vi "RtdeGetLatestOutputValues.vi"(8 "Rtde":refnum<k24>, 11 "error in":errorcluster) -> (0 "Data":T1, 3 "error out":errorcluster)   [LabVIEW 2015, in "UnderAutomation.UniversalRobots.lvlib"]
uses:
  UnderAutomation.UniversalRobots.lvlib
  C:/Users/fg/Documents/UniversalRobots.vi/LabVIEW_2024/UnderAutomation.UniversalRobots/lib/UnderAutomation.UniversalRobots.dll
  LabVIEW_2024/UnderAutomation.UniversalRobots/lib/UnderAutomation.UniversalRobots.dll
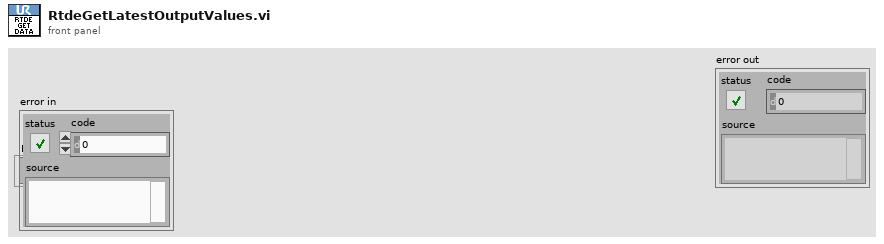
[diagram p1: front panel]
types:
  T1 = cluster{"ActualCurrent":cluster{"Base":dbl, "Elbow":dbl, "Shoulder":dbl, "Wrist1":dbl, "Wrist2":dbl, "Wrist3":dbl}, "ActualDigitalInputBits":u64, "ActualDigitalOutputBits":u64, "ActualExecutionTime":dbl, "ActualJointVoltage":cluster{"Base":dbl, "Elbow":dbl, "Shoulder":dbl, "Wrist1":dbl, "Wrist2":dbl, "Wrist3":dbl}, "ActualMainVoltage":dbl, "ActualMomentum":dbl, "ActualQ":cluster{"Base":dbl, "Elbow":dbl, "Shoulder":dbl, "Wrist1":dbl, "Wrist2":dbl, "Wrist3":dbl}, "ActualQd":cluster{"Base":dbl, "Elbow":dbl, "Shoulder":dbl, "Wrist1":dbl, "Wrist2":dbl, "Wrist3":dbl}, "ActualRobotCurrent":dbl, "ActualRobotVoltage":dbl, "ActualTcpForce":cluster{"X":dbl, "Y":dbl, "Z":dbl, "Rx":dbl, "Ry":dbl, "Rz":dbl}, "ActualTcpPose":cluster{"X":dbl, "Y":dbl, "Z":dbl, "Rx":dbl, "Ry":dbl, "Rz":dbl}, "ActualTcpSpeed":cluster{"X":dbl, "Y":dbl, "Z":dbl, "Rx":dbl, "Ry":dbl, "Rz":dbl}, "ActualToolAccelerometer":cluster{"X":dbl, "Y":dbl, "Z":dbl}, "AnalogIOTypes":u32, "ElbowPosition":cluster{"X":dbl, "Y":dbl, "Z":dbl}, "ElbowVelocity":cluster{"X":dbl, "Y":dbl, "Z":dbl}, "Euromap67_24VCurrent":dbl, "Euromap67_24VVoltage":dbl, "Euromap67InputBits":u32, "Euromap67OutputBits":u32, "FTRawWrench":cluster{"X":dbl, "Y":dbl, "Z":dbl, "Rx":dbl, "Ry":dbl, "Rz":dbl}, "InputBitRegisters":cluster{"X64":bool, "X65":bool, "X66":bool, "X67":bool, "X68":bool, "X69":bool, "X70":bool, "X71":bool, "X72":bool, "X73":bool, "X74":bool, "X75":bool, "X76":bool, "X77":bool, "X78":bool, "X79":bool, "X80":bool, "X81":bool, "X82":bool, "X83":bool, "X84":bool, "X85":bool, "X86":bool, "X87":bool, "X88":bool, "X89":bool, "X90":bool, "X91":bool, "X92":bool, "X93":bool, "X94":bool, "X95":bool, "X96":bool, "X97":bool, "X98":bool, "X99":bool, "X100":bool, "X101":bool, "X102":bool, "X103":bool, "X104":bool, "X105":bool, "X106":bool, "X107":bool, "X108":bool, "X109":bool, "X110":bool, "X111":bool, "X112":bool, "X113":bool, "X114":bool, "X115":bool, "X116":bool, "X117":bool, "X118":bool, "X119":bool, "X120":bool, "X121":bool, "X122":bool, "X123":bool, "X124":bool, "X125":bool, "X126":bool, "X127":bool}, "InputBitRegisters0To31":u32, "InputBitRegisters32To63":u32, "InputDoubleRegisters":cluster{"X0":dbl, "X1":dbl, "X2":dbl, "X3":dbl, "X4":dbl, "X5":dbl, "X6":dbl, "X7":dbl, "X8":dbl, "X9":dbl, "X10":dbl, "X11":dbl, "X12":dbl, "X13":dbl, "X14":dbl, "X15":dbl, "X16":dbl, "X17":dbl, "X18":dbl, "X19":dbl, "X20":dbl, "X21":dbl, "X22":dbl, "X23":dbl, "X24":dbl, "X25":dbl, "X26":dbl, "X27":dbl, "X28":dbl, "X29":dbl, "X30":dbl, "X31":dbl, "X32":dbl, "X33":dbl, "X34":dbl, "X35":dbl, "X36":dbl, "X37":dbl, "X38":dbl, "X39":dbl, "X40":dbl, "X41":dbl, "X42":dbl, "X43":dbl, "X44":dbl, "X45":dbl, "X46":dbl, "X47":dbl}, "InputIntRegisters":cluster{"X0":i32, "X1":i32, "X2":i32, "X3":i32, "X4":i32, "X5":i32, "X6":i32, "X7":i32, "X8":i32, "X9":i32, "X10":i32, "X11":i32, "X12":i32, "X13":i32, "X14":i32, "X15":i32, "X16":i32, "X17":i32, "X18":i32, "X19":i32, "X20":i32, "X21":i32, "X22":i32, "X23":i32, "X24":i32, "X25":i32, "X26":i32, "X27":i32, "X28":i32, "X29":i32, "X30":i32, "X31":i32, "X32":i32, "X33":i32, "X34":i32, "X35":i32, "X36":i32, "X37":i32, "X38":i32, "X39":i32, "X40":i32, "X41":i32, "X42":i32, "X43":i32, "X44":i32, "X45":i32, "X46":i32, "X47":i32}, "IOCurrent":dbl, "JointControlOutput":cluster{"Base":dbl, "Elbow":dbl, "Shoulder":dbl, "Wrist1":dbl, "Wrist2":dbl, "Wrist3":dbl}, "JointMode":cluster{"Base":i32, "Elbow":i32, "Shoulder":i32, "Wrist1":i32, "Wrist2":i32, "Wrist3":i32}, "JointTemperatures":cluster{"Base":dbl, "Elbow":dbl, "Shoulder":dbl, "Wrist1":dbl, "Wrist2":dbl, "Wrist3":dbl}, "OutputBitRegisters":cluster{"X64":bool, "X65":bool, "X66":bool, "X67":bool, "X68":bool, "X69":bool, "X70":bool, "X71":bool, "X72":bool, "X73":bool, "X74":bool, "X75":bool, "X76":bool, "X77":bool, "X78":bool, "X79":bool, "X80":bool, "X81":bool, "X82":bool, "X83":bool, "X84":bool, "X85":bool, "X86":bool, "X87":bool, "X88":bool, "X89":bool, "X90":bool, "X91":bool, "X92":bool, "X93":bool, "X94":bool, "X95":bool, "X96":bool, "X97":bool, "X98":bool, "X99":bool, "X100":bool, "X101":bool, "X102":bool, "X103":bool, "X104":bool, "X105":bool, "X106":bool, "X107":bool, "X108":bool, "X109":bool, "X110":bool, "X111":bool, "X112":bool, "X113":bool, "X114":bool, "X115":bool, "X116":bool, "X117":bool, "X118":bool, "X119":bool, "X120":bool, "X121":bool, "X122":bool, "X123":bool, "X124":bool, "X125":bool, "X126":bool, "X127":bool}, "OutputBitRegisters0To31":u32, "OutputBitRegisters32To63":u32, "OutputDoubleRegisters":cluster{"X0":dbl, "X1":dbl, "X2":dbl, "X3":dbl, "X4":dbl, "X5":dbl, "X6":dbl, "X7":dbl, "X8":dbl, "X9":dbl, "X10":dbl, "X11":dbl, "X12":dbl, "X13":dbl, "X14":dbl, "X15":dbl, "X16":dbl, "X17":dbl, "X18":dbl, "X19":dbl, "X20":dbl, "X21":dbl, "X22":dbl, "X23":dbl, "X24":dbl, "X25":dbl, "X26":dbl, "X27":dbl, "X28":dbl, "X29":dbl, "X30":dbl, "X31":dbl, "X32":dbl, "X33":dbl, "X34":dbl, "X35":dbl, "X36":dbl, "X37":dbl, "X38":dbl, "X39":dbl, "X40":dbl, "X41":dbl, "X42":dbl, "X43":dbl, "X44":dbl, "X45":dbl, "X46":dbl, "X47":dbl}, "OutputIntRegisters":cluster{"X0":i32, "X1":i32, "X2":i32, "X3":i32, "X4":i32, "X5":i32, "X6":i32, "X7":i32, "X8":i32, "X9":i32, "X10":i32, "X11":i32, "X12":i32, "X13":i32, "X14":i32, "X15":i32, "X16":i32, "X17":i32, "X18":i32, "X19":i32, "X20":i32, "X21":i32, "X22":i32, "X23":i32, "X24":i32, "X25":i32, "X26":i32, "X27":i32, "X28":i32, "X29":i32, "X30":i32, "X31":i32, "X32":i32, "X33":i32, "X34":i32, "X35":i32, "X36":i32, "X37":i32, "X38":i32, "X39":i32, "X40":i32, "X41":i32, "X42":i32, "X43":i32, "X44":i32, "X45":i32, "X46":i32, "X47":i32}, "Payload":dbl, "PayloadCOG":cluster{"X":dbl, "Y":dbl, "Z":dbl}, "PayloadInertia":cluster{"X":dbl, "Y":dbl, "Z":dbl, "Rx":dbl, "Ry":dbl, "Rz":dbl}, "RobotMode":i32, "RobotStatusBits":u32, "RuntimeState":u32, "SafetyMode":i32, "SafetyStatus":i32, "SafetyStatusBits":u32, "ScriptControlLine":u32, "SpeedScaling":dbl, "StandardAnalogInput0":dbl, "StandardAnalogInput1":dbl, "StandardAnalogOutput0":dbl, "StandardAnalogOutput1":dbl, "TargetCurrent":cluster{"Base":dbl, "Elbow":dbl, "Shoulder":dbl, "Wrist1":dbl, "Wrist2":dbl, "Wrist3":dbl}, "TargetMoment":cluster{"Base":dbl, "Elbow":dbl, "Shoulder":dbl, "Wrist1":dbl, "Wrist2":dbl, "Wrist3":dbl}, "TargetQ":cluster{"Base":dbl, "Elbow":dbl, "Shoulder":dbl, "Wrist1":dbl, "Wrist2":dbl, "Wrist3":dbl}, "TargetQd":cluster{"Base":dbl, "Elbow":dbl, "Shoulder":dbl, "Wrist1":dbl, "Wrist2":dbl, "Wrist3":dbl}, "TargetQdd":cluster{"Base":dbl, "Elbow":dbl, "Shoulder":dbl, "Wrist1":dbl, "Wrist2":dbl, "Wrist3":dbl}, "TargetSpeedFraction":dbl, "TargetTcpPose":cluster{"X":dbl, "Y":dbl, "Z":dbl, "Rx":dbl, "Ry":dbl, "Rz":dbl}, "TargetTcpSpeed":cluster{"X":dbl, "Y":dbl, "Z":dbl, "Rx":dbl, "Ry":dbl, "Rz":dbl}, "TcpForceScalar":dbl, "Timestamp":dbl, "ToolAnalogInput0":dbl, "ToolAnalogInput1":dbl, "ToolAnalogInputTypes":u32, "ToolDigitalOutput0mode":u8, "ToolDigitalOutput1Mode":u8, "ToolMode":u32, "ToolOutputCurrent":dbl, "ToolOutputMode":u8, "ToolOutputVoltage":i32, "ToolTemperature":dbl}
  T2 = cluster{"Base":dbl, "Elbow":dbl, "Shoulder":dbl, "Wrist1":dbl, "Wrist2":dbl, "Wrist3":dbl}
  T3 = cluster{"X":dbl, "Y":dbl, "Z":dbl, "Rx":dbl, "Ry":dbl, "Rz":dbl}
  T4 = cluster{"X64":bool, "X65":bool, "X66":bool, "X67":bool, "X68":bool, "X69":bool, "X70":bool, "X71":bool, "X72":bool, "X73":bool, "X74":bool, "X75":bool, "X76":bool, "X77":bool, "X78":bool, "X79":bool, "X80":bool, "X81":bool, "X82":bool, "X83":bool, "X84":bool, "X85":bool, "X86":bool, "X87":bool, "X88":bool, "X89":bool, "X90":bool, "X91":bool, "X92":bool, "X93":bool, "X94":bool, "X95":bool, "X96":bool, "X97":bool, "X98":bool, "X99":bool, "X100":bool, "X101":bool, "X102":bool, "X103":bool, "X104":bool, "X105":bool, "X106":bool, "X107":bool, "X108":bool, "X109":bool, "X110":bool, "X111":bool, "X112":bool, "X113":bool, "X114":bool, "X115":bool, "X116":bool, "X117":bool, "X118":bool, "X119":bool, "X120":bool, "X121":bool, "X122":bool, "X123":bool, "X124":bool, "X125":bool, "X126":bool, "X127":bool}
  T5 = cluster{"X0":dbl, "X1":dbl, "X2":dbl, "X3":dbl, "X4":dbl, "X5":dbl, "X6":dbl, "X7":dbl, "X8":dbl, "X9":dbl, "X10":dbl, "X11":dbl, "X12":dbl, "X13":dbl, "X14":dbl, "X15":dbl, "X16":dbl, "X17":dbl, "X18":dbl, "X19":dbl, "X20":dbl, "X21":dbl, "X22":dbl, "X23":dbl, "X24":dbl, "X25":dbl, "X26":dbl, "X27":dbl, "X28":dbl, "X29":dbl, "X30":dbl, "X31":dbl, "X32":dbl, "X33":dbl, "X34":dbl, "X35":dbl, "X36":dbl, "X37":dbl, "X38":dbl, "X39":dbl, "X40":dbl, "X41":dbl, "X42":dbl, "X43":dbl, "X44":dbl, "X45":dbl, "X46":dbl, "X47":dbl}
  T6 = cluster{"Base":i32, "Elbow":i32, "Shoulder":i32, "Wrist1":i32, "Wrist2":i32, "Wrist3":i32}
  T7 = cluster{"X0":i32, "X1":i32, "X2":i32, "X3":i32, "X4":i32, "X5":i32, "X6":i32, "X7":i32, "X8":i32, "X9":i32, "X10":i32, "X11":i32, "X12":i32, "X13":i32, "X14":i32, "X15":i32, "X16":i32, "X17":i32, "X18":i32, "X19":i32, "X20":i32, "X21":i32, "X22":i32, "X23":i32, "X24":i32, "X25":i32, "X26":i32, "X27":i32, "X28":i32, "X29":i32, "X30":i32, "X31":i32, "X32":i32, "X33":i32, "X34":i32, "X35":i32, "X36":i32, "X37":i32, "X38":i32, "X39":i32, "X40":i32, "X41":i32, "X42":i32, "X43":i32, "X44":i32, "X45":i32, "X46":i32, "X47":i32}
  T8 = cluster{cluster{"Base":dbl, "Elbow":dbl, "Shoulder":dbl, "Wrist1":dbl, "Wrist2":dbl, "Wrist3":dbl}, "ActualDigitalInputBits":u64, "ActualDigitalOutputBits":u64, "ActualExecutionTime":dbl, cluster{"Base":dbl, "Elbow":dbl, "Shoulder":dbl, "Wrist1":dbl, "Wrist2":dbl, "Wrist3":dbl}, "ActualMainVoltage":dbl, "ActualMomentum":dbl, cluster{"Base":dbl, "Elbow":dbl, "Shoulder":dbl, "Wrist1":dbl, "Wrist2":dbl, "Wrist3":dbl}, cluster{"Base":dbl, "Elbow":dbl, "Shoulder":dbl, "Wrist1":dbl, "Wrist2":dbl, "Wrist3":dbl}, "ActualRobotCurrent":dbl, "ActualRobotVoltage":dbl, cluster{"X":dbl, "Y":dbl, "Z":dbl, "Rx":dbl, "Ry":dbl, "Rz":dbl}, cluster{"X":dbl, "Y":dbl, "Z":dbl, "Rx":dbl, "Ry":dbl, "Rz":dbl}, cluster{"X":dbl, "Y":dbl, "Z":dbl, "Rx":dbl, "Ry":dbl, "Rz":dbl}, cluster{"X":dbl, "Y":dbl, "Z":dbl}, "AnalogIOTypes":u32, cluster{"X":dbl, "Y":dbl, "Z":dbl}, cluster{"X":dbl, "Y":dbl, "Z":dbl}, "Euromap67_24VCurrent":dbl, "Euromap67_24VVoltage":dbl, "Euromap67InputBits":u32, "Euromap67OutputBits":u32, cluster{"X":dbl, "Y":dbl, "Z":dbl, "Rx":dbl, "Ry":dbl, "Rz":dbl}, cluster{"X64":bool, "X65":bool, "X66":bool, "X67":bool, "X68":bool, "X69":bool, "X70":bool, "X71":bool, "X72":bool, "X73":bool, "X74":bool, "X75":bool, "X76":bool, "X77":bool, "X78":bool, "X79":bool, "X80":bool, "X81":bool, "X82":bool, "X83":bool, "X84":bool, "X85":bool, "X86":bool, "X87":bool, "X88":bool, "X89":bool, "X90":bool, "X91":bool, "X92":bool, "X93":bool, "X94":bool, "X95":bool, "X96":bool, "X97":bool, "X98":bool, "X99":bool, "X100":bool, "X101":bool, "X102":bool, "X103":bool, "X104":bool, "X105":bool, "X106":bool, "X107":bool, "X108":bool, "X109":bool, "X110":bool, "X111":bool, "X112":bool, "X113":bool, "X114":bool, "X115":bool, "X116":bool, "X117":bool, "X118":bool, "X119":bool, "X120":bool, "X121":bool, "X122":bool, "X123":bool, "X124":bool, "X125":bool, "X126":bool, "X127":bool}, "InputBitRegisters0To31":u32, "InputBitRegisters32To63":u32, cluster{"X0":dbl, "X1":dbl, "X2":dbl, "X3":dbl, "X4":dbl, "X5":dbl, "X6":dbl, "X7":dbl, "X8":dbl, "X9":dbl, "X10":dbl, "X11":dbl, "X12":dbl, "X13":dbl, "X14":dbl, "X15":dbl, "X16":dbl, "X17":dbl, "X18":dbl, "X19":dbl, "X20":dbl, "X21":dbl, "X22":dbl, "X23":dbl, "X24":dbl, "X25":dbl, "X26":dbl, "X27":dbl, "X28":dbl, "X29":dbl, "X30":dbl, "X31":dbl, "X32":dbl, "X33":dbl, "X34":dbl, "X35":dbl, "X36":dbl, "X37":dbl, "X38":dbl, "X39":dbl, "X40":dbl, "X41":dbl, "X42":dbl, "X43":dbl, "X44":dbl, "X45":dbl, "X46":dbl, "X47":dbl}, cluster{"X0":i32, "X1":i32, "X2":i32, "X3":i32, "X4":i32, "X5":i32, "X6":i32, "X7":i32, "X8":i32, "X9":i32, "X10":i32, "X11":i32, "X12":i32, "X13":i32, "X14":i32, "X15":i32, "X16":i32, "X17":i32, "X18":i32, "X19":i32, "X20":i32, "X21":i32, "X22":i32, "X23":i32, "X24":i32, "X25":i32, "X26":i32, "X27":i32, "X28":i32, "X29":i32, "X30":i32, "X31":i32, "X32":i32, "X33":i32, "X34":i32, "X35":i32, "X36":i32, "X37":i32, "X38":i32, "X39":i32, "X40":i32, "X41":i32, "X42":i32, "X43":i32, "X44":i32, "X45":i32, "X46":i32, "X47":i32}, "IOCurrent":dbl, cluster{"Base":dbl, "Elbow":dbl, "Shoulder":dbl, "Wrist1":dbl, "Wrist2":dbl, "Wrist3":dbl}, cluster{"Base":i32, "Elbow":i32, "Shoulder":i32, "Wrist1":i32, "Wrist2":i32, "Wrist3":i32}, cluster{"Base":dbl, "Elbow":dbl, "Shoulder":dbl, "Wrist1":dbl, "Wrist2":dbl, "Wrist3":dbl}, cluster{"X64":bool, "X65":bool, "X66":bool, "X67":bool, "X68":bool, "X69":bool, "X70":bool, "X71":bool, "X72":bool, "X73":bool, "X74":bool, "X75":bool, "X76":bool, "X77":bool, "X78":bool, "X79":bool, "X80":bool, "X81":bool, "X82":bool, "X83":bool, "X84":bool, "X85":bool, "X86":bool, "X87":bool, "X88":bool, "X89":bool, "X90":bool, "X91":bool, "X92":bool, "X93":bool, "X94":bool, "X95":bool, "X96":bool, "X97":bool, "X98":bool, "X99":bool, "X100":bool, "X101":bool, "X102":bool, "X103":bool, "X104":bool, "X105":bool, "X106":bool, "X107":bool, "X108":bool, "X109":bool, "X110":bool, "X111":bool, "X112":bool, "X113":bool, "X114":bool, "X115":bool, "X116":bool, "X117":bool, "X118":bool, "X119":bool, "X120":bool, "X121":bool, "X122":bool, "X123":bool, "X124":bool, "X125":bool, "X126":bool, "X127":bool}, "OutputBitRegisters0To31":u32, "OutputBitRegisters32To63":u32, cluster{"X0":dbl, "X1":dbl, "X2":dbl, "X3":dbl, "X4":dbl, "X5":dbl, "X6":dbl, "X7":dbl, "X8":dbl, "X9":dbl, "X10":dbl, "X11":dbl, "X12":dbl, "X13":dbl, "X14":dbl, "X15":dbl, "X16":dbl, "X17":dbl, "X18":dbl, "X19":dbl, "X20":dbl, "X21":dbl, "X22":dbl, "X23":dbl, "X24":dbl, "X25":dbl, "X26":dbl, "X27":dbl, "X28":dbl, "X29":dbl, "X30":dbl, "X31":dbl, "X32":dbl, "X33":dbl, "X34":dbl, "X35":dbl, "X36":dbl, "X37":dbl, "X38":dbl, "X39":dbl, "X40":dbl, "X41":dbl, "X42":dbl, "X43":dbl, "X44":dbl, "X45":dbl, "X46":dbl, "X47":dbl}, cluster{"X0":i32, "X1":i32, "X2":i32, "X3":i32, "X4":i32, "X5":i32, "X6":i32, "X7":i32, "X8":i32, "X9":i32, "X10":i32, "X11":i32, "X12":i32, "X13":i32, "X14":i32, "X15":i32, "X16":i32, "X17":i32, "X18":i32, "X19":i32, "X20":i32, "X21":i32, "X22":i32, "X23":i32, "X24":i32, "X25":i32, "X26":i32, "X27":i32, "X28":i32, "X29":i32, "X30":i32, "X31":i32, "X32":i32, "X33":i32, "X34":i32, "X35":i32, "X36":i32, "X37":i32, "X38":i32, "X39":i32, "X40":i32, "X41":i32, "X42":i32, "X43":i32, "X44":i32, "X45":i32, "X46":i32, "X47":i32}, "Payload":dbl, cluster{"X":dbl, "Y":dbl, "Z":dbl}, cluster{"X":dbl, "Y":dbl, "Z":dbl, "Rx":dbl, "Ry":dbl, "Rz":dbl}, "RobotMode":i32, "RobotStatusBits":u32, "RuntimeState":u32, "SafetyMode":i32, "SafetyStatus":i32, "SafetyStatusBits":u32, "ScriptControlLine":u32, "SpeedScaling":dbl, "StandardAnalogInput0":dbl, "StandardAnalogInput1":dbl, "StandardAnalogOutput0":dbl, "StandardAnalogOutput1":dbl, cluster{"Base":dbl, "Elbow":dbl, "Shoulder":dbl, "Wrist1":dbl, "Wrist2":dbl, "Wrist3":dbl}, cluster{"Base":dbl, "Elbow":dbl, "Shoulder":dbl, "Wrist1":dbl, "Wrist2":dbl, "Wrist3":dbl}, cluster{"Base":dbl, "Elbow":dbl, "Shoulder":dbl, "Wrist1":dbl, "Wrist2":dbl, "Wrist3":dbl}, cluster{"Base":dbl, "Elbow":dbl, "Shoulder":dbl, "Wrist1":dbl, "Wrist2":dbl, "Wrist3":dbl}, cluster{"Base":dbl, "Elbow":dbl, "Shoulder":dbl, "Wrist1":dbl, "Wrist2":dbl, "Wrist3":dbl}, "TargetSpeedFraction":dbl, cluster{"X":dbl, "Y":dbl, "Z":dbl, "Rx":dbl, "Ry":dbl, "Rz":dbl}, cluster{"X":dbl, "Y":dbl, "Z":dbl, "Rx":dbl, "Ry":dbl, "Rz":dbl}, "TcpForceScalar":dbl, "Timestamp":dbl, "ToolAnalogInput0":dbl, "ToolAnalogInput1":dbl, "ToolAnalogInputTypes":u32, "ToolDigitalOutput0mode":u8, "ToolDigitalOutput1Mode":u8, "ToolMode":u32, "ToolOutputCurrent":dbl, "ToolOutputMode":u8, "ToolOutputVoltage":i32, "ToolTemperature":dbl}
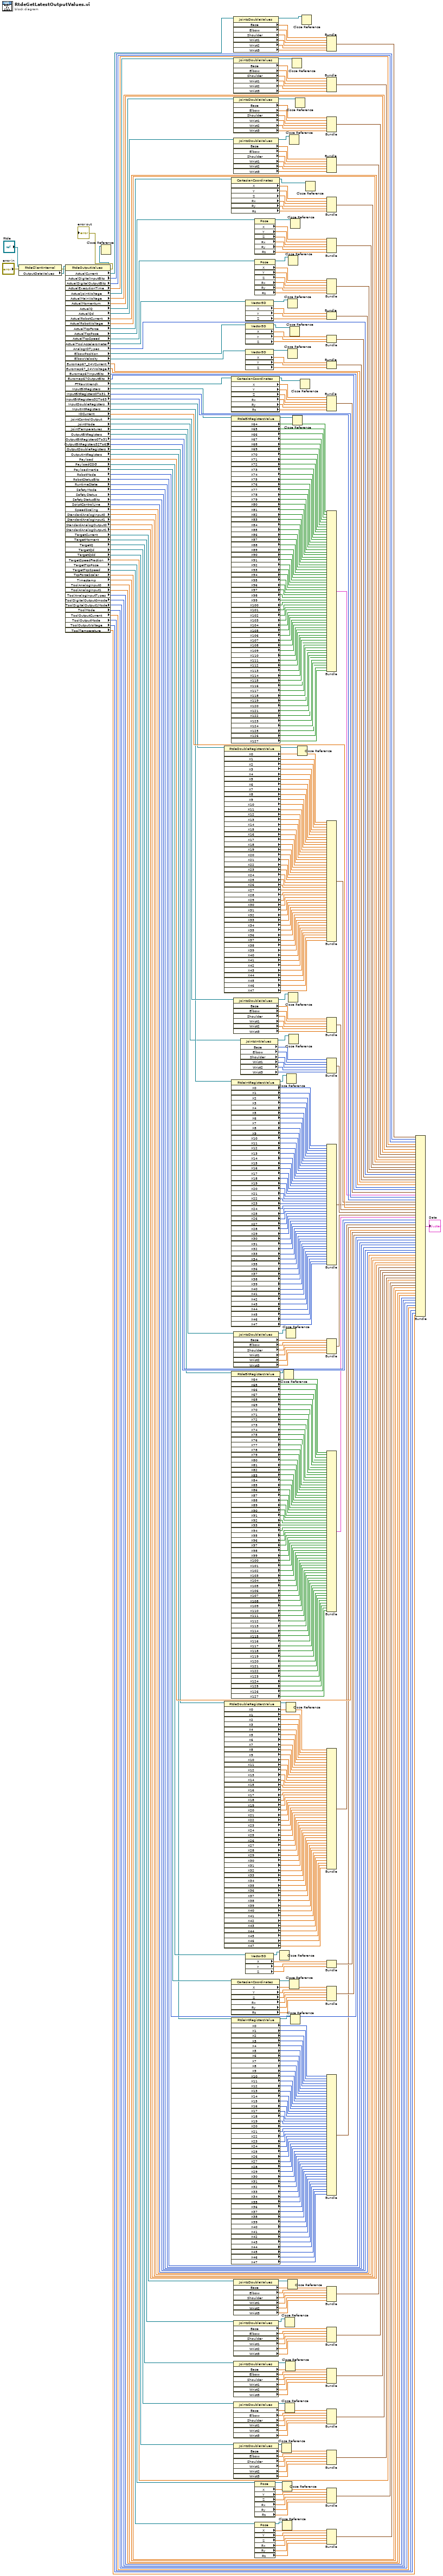
[diagram p0: block diagram]
diagram:
  n1 = property class="RtdeClientInternal"(reference="Rtde", error in="error in") -> (error out=w31:errorcluster, "OutputDataValues"=w32:refnum<k24>)  [unwired: 1 out]
  n2 = property on="Property Node" class="RtdeOutputValues"(reference=w32, error in=w31) -> (reference out=w1:refnum<k24>, error out=→"error out":errorcluster, "ActualCurrent"=w34:refnum<k24>, "ActualDigitalInputBits"=w156:u64, "ActualDigitalOutputBits"=w157:u64, "ActualExecutionTime"=w158:dbl, "ActualJointVoltage"=w41:refnum<k24>, "ActualMainVoltage"=w160:dbl, "ActualMomentum"=w161:dbl, "ActualQ"=w113:refnum<k24>, "ActualQd"=w120:refnum<k24>, "ActualRobotCurrent"=w164:dbl, "ActualRobotVoltage"=w165:dbl, "ActualTcpForce"=w179:refnum<k24>, "ActualTcpPose"=w166:refnum<k24>, "ActualTcpSpeed"=w188:refnum<k24>, "ActualToolAccelerometer"=w190:refnum<k24>, "AnalogIOTypes"=w195:u32, "ElbowPosition"=w196:refnum<k24>, "ElbowVelocity"=w201:refnum<k24>, "Euromap67_24VCurrent"=w206:dbl, "Euromap67_24VVoltage"=w207:dbl, "Euromap67InputBits"=w208:u32, "Euromap67OutputBits"=w209:u32, "FTRawWrench"=w216:refnum<k24>, "InputBitRegisters"=w282:refnum<k24>, "InputBitRegisters0To31"=w334:u32, "InputBitRegisters32To63"=w333:u32, "InputDoubleRegisters"=w284:refnum<k24>, "InputIntRegisters"=w384:refnum<k24>, "IOCurrent"=w386:dbl, "JointControlOutput"=w393:refnum<k24>, "JointMode"=w127:refnum<k24>, "JointTemperatures"=w402:refnum<k24>, "OutputBitRegisters"=w42:refnum<k24>, "OutputBitRegisters0To31"=w405:u32, "OutputBitRegisters32To63"=w406:u32, "OutputDoubleRegisters"=w455:refnum<k24>, "OutputIntRegisters"=w505:refnum<k24>, "Payload"=w511:dbl, "PayloadCOG"=w510:refnum<k24>, "PayloadInertia"=w519:refnum<k24>, "RobotMode"=w521:i32, "RobotStatusBits"=w522:u32, "RuntimeState"=w523:u32, "SafetyMode"=w524:i32, "SafetyStatus"=w525:i32, "SafetyStatusBits"=w526:u32, "ScriptControlLine"=w527:u32, "SpeedScaling"=w528:dbl, "StandardAnalogInput0"=w529:dbl, "StandardAnalogInput1"=w530:dbl, "StandardAnalogOutput0"=w531:dbl, "StandardAnalogOutput1"=w532:dbl, "TargetCurrent"=w545:refnum<k24>, "TargetMoment"=w546:refnum<k24>, "TargetQ"=w152:refnum<k24>, "TargetQd"=w153:refnum<k24>, "TargetQdd"=w154:refnum<k24>, "TargetSpeedFraction"=w552:dbl, "TargetTcpPose"=w565:refnum<k24>, "TargetTcpSpeed"=w566:refnum<k24>, "TcpForceScalar"=w569:dbl, "Timestamp"=w570:dbl, "ToolAnalogInput0"=w571:dbl, "ToolAnalogInput1"=w572:dbl, "ToolAnalogInputTypes"=w573:u32, "ToolDigitalOutput0mode"=w574:u8, "ToolDigitalOutput1Mode"=w575:u8, "ToolMode"=w576:u32, "ToolOutputCurrent"=w577:dbl, "ToolOutputMode"=w578:u8, "ToolOutputVoltage"=w579:i32, "ToolTemperature"=w580:dbl)
  n3 = Close Reference(reference=w1) -> ()  [unwired: 1 in, 1 out]
  n4 = property class="RtdeDoubleRegistersValue"(reference=w284) -> (reference out=w18:refnum<k24>, "X0"=w285:dbl, "X1"=w286:dbl, "X2"=w287:dbl, "X3"=w288:dbl, "X4"=w289:dbl, "X5"=w290:dbl, "X6"=w291:dbl, "X7"=w292:dbl, "X8"=w293:dbl, "X9"=w294:dbl, "X10"=w295:dbl, "X11"=w296:dbl, "X12"=w297:dbl, "X13"=w298:dbl, "X14"=w299:dbl, "X15"=w300:dbl, "X16"=w301:dbl, "X17"=w302:dbl, "X18"=w303:dbl, "X19"=w304:dbl, "X20"=w305:dbl, "X21"=w306:dbl, "X22"=w307:dbl, "X23"=w308:dbl, "X24"=w309:dbl, "X25"=w310:dbl, "X26"=w311:dbl, "X27"=w312:dbl, "X28"=w313:dbl, "X29"=w314:dbl, "X30"=w315:dbl, "X31"=w316:dbl, "X32"=w317:dbl, "X33"=w318:dbl, "X34"=w319:dbl, "X35"=w320:dbl, "X36"=w321:dbl, "X37"=w322:dbl, "X38"=w323:dbl, "X39"=w324:dbl, "X40"=w325:dbl, "X41"=w326:dbl, "X42"=w327:dbl, "X43"=w328:dbl, "X44"=w329:dbl, "X45"=w330:dbl, "X46"=w331:dbl, "X47"=w332:dbl)  [unwired: 1 in, 1 out]
  n5 = property class="RtdeDoubleRegistersValue"(reference=w455) -> (reference out=w12:refnum<k24>, "X0"=w407:dbl, "X1"=w408:dbl, "X2"=w409:dbl, "X3"=w410:dbl, "X4"=w411:dbl, "X5"=w412:dbl, "X6"=w413:dbl, "X7"=w414:dbl, "X8"=w415:dbl, "X9"=w416:dbl, "X10"=w417:dbl, "X11"=w418:dbl, "X12"=w419:dbl, "X13"=w420:dbl, "X14"=w421:dbl, "X15"=w422:dbl, "X16"=w423:dbl, "X17"=w424:dbl, "X18"=w425:dbl, "X19"=w426:dbl, "X20"=w427:dbl, "X21"=w428:dbl, "X22"=w429:dbl, "X23"=w430:dbl, "X24"=w431:dbl, "X25"=w432:dbl, "X26"=w433:dbl, "X27"=w434:dbl, "X28"=w435:dbl, "X29"=w436:dbl, "X30"=w437:dbl, "X31"=w438:dbl, "X32"=w439:dbl, "X33"=w440:dbl, "X34"=w441:dbl, "X35"=w442:dbl, "X36"=w443:dbl, "X37"=w444:dbl, "X38"=w445:dbl, "X39"=w446:dbl, "X40"=w447:dbl, "X41"=w448:dbl, "X42"=w449:dbl, "X43"=w450:dbl, "X44"=w451:dbl, "X45"=w452:dbl, "X46"=w453:dbl, "X47"=w454:dbl)  [unwired: 1 in, 1 out]
  n6 = property class="CartesianCoordinates"(reference=w179) -> (reference out=w26:refnum<k24>, "X"=w178:dbl, "Y"=w177:dbl, "Z"=w176:dbl, "Rx"=w175:dbl, "Ry"=w174:dbl, "Rz"=w173:dbl)  [unwired: 1 in, 1 out]
  n7 = property class="CartesianCoordinates"(reference=w216) -> (reference out=w20:refnum<k24>, "X"=w210:dbl, "Y"=w211:dbl, "Z"=w212:dbl, "Rx"=w213:dbl, "Ry"=w214:dbl, "Rz"=w215:dbl)  [unwired: 1 in, 1 out]
  n8 = property class="CartesianCoordinates"(reference=w519) -> (reference out=w10:refnum<k24>, "X"=w513:dbl, "Y"=w514:dbl, "Z"=w515:dbl, "Rx"=w516:dbl, "Ry"=w517:dbl, "Rz"=w518:dbl)  [unwired: 1 in, 1 out]
  n9 = property class="RtdeBitRegistersValue"(reference=w282) -> (reference out=w19:refnum<k24>, "X64"=w281:bool, "X65"=w280:bool, "X66"=w279:bool, "X67"=w278:bool, "X68"=w277:bool, "X69"=w276:bool, "X70"=w275:bool, "X71"=w274:bool, "X72"=w273:bool, "X73"=w272:bool, "X74"=w271:bool, "X75"=w270:bool, "X76"=w269:bool, "X77"=w268:bool, "X78"=w267:bool, "X79"=w266:bool, "X80"=w265:bool, "X81"=w264:bool, "X82"=w263:bool, "X83"=w262:bool, "X84"=w261:bool, "X85"=w260:bool, "X86"=w259:bool, "X87"=w258:bool, "X88"=w257:bool, "X89"=w256:bool, "X90"=w255:bool, "X91"=w254:bool, "X92"=w253:bool, "X93"=w252:bool, "X94"=w251:bool, "X95"=w250:bool, "X96"=w249:bool, "X97"=w248:bool, "X98"=w247:bool, "X99"=w246:bool, "X100"=w245:bool, "X101"=w244:bool, "X102"=w243:bool, "X103"=w242:bool, "X104"=w241:bool, "X105"=w240:bool, "X106"=w239:bool, "X107"=w238:bool, "X108"=w237:bool, "X109"=w236:bool, "X110"=w235:bool, "X111"=w234:bool, "X112"=w233:bool, "X113"=w232:bool, "X114"=w231:bool, "X115"=w230:bool, "X116"=w229:bool, "X117"=w228:bool, "X118"=w227:bool, "X119"=w226:bool, "X120"=w225:bool, "X121"=w224:bool, "X122"=w223:bool, "X123"=w222:bool, "X124"=w221:bool, "X125"=w220:bool, "X126"=w219:bool, "X127"=w218:bool)  [unwired: 1 in, 1 out]
  n10 = property class="RtdeIntRegistersValue"(reference=w384) -> (reference out=w15:refnum<k24>, "X0"=w336:i32, "X1"=w337:i32, "X2"=w338:i32, "X3"=w339:i32, "X4"=w340:i32, "X5"=w341:i32, "X6"=w342:i32, "X7"=w343:i32, "X8"=w344:i32, "X9"=w345:i32, "X10"=w346:i32, "X11"=w347:i32, "X12"=w348:i32, "X13"=w349:i32, "X14"=w350:i32, "X15"=w351:i32, "X16"=w352:i32, "X17"=w353:i32, "X18"=w354:i32, "X19"=w355:i32, "X20"=w356:i32, "X21"=w357:i32, "X22"=w358:i32, "X23"=w359:i32, "X24"=w360:i32, "X25"=w361:i32, "X26"=w362:i32, "X27"=w363:i32, "X28"=w364:i32, "X29"=w365:i32, "X30"=w366:i32, "X31"=w367:i32, "X32"=w368:i32, "X33"=w369:i32, "X34"=w370:i32, "X35"=w371:i32, "X36"=w372:i32, "X37"=w373:i32, "X38"=w374:i32, "X39"=w375:i32, "X40"=w376:i32, "X41"=w377:i32, "X42"=w378:i32, "X43"=w379:i32, "X44"=w380:i32, "X45"=w381:i32, "X46"=w382:i32, "X47"=w383:i32)  [unwired: 1 in, 1 out]
  n11 = property class="RtdeBitRegistersValue"(reference=w42) -> (reference out=w13:refnum<k24>, "X64"=w43:bool, "X65"=w44:bool, "X66"=w45:bool, "X67"=w46:bool, "X68"=w47:bool, "X69"=w48:bool, "X70"=w49:bool, "X71"=w50:bool, "X72"=w51:bool, "X73"=w52:bool, "X74"=w53:bool, "X75"=w54:bool, "X76"=w55:bool, "X77"=w56:bool, "X78"=w57:bool, "X79"=w58:bool, "X80"=w59:bool, "X81"=w60:bool, "X82"=w61:bool, "X83"=w62:bool, "X84"=w63:bool, "X85"=w64:bool, "X86"=w65:bool, "X87"=w66:bool, "X88"=w67:bool, "X89"=w68:bool, "X90"=w69:bool, "X91"=w70:bool, "X92"=w71:bool, "X93"=w72:bool, "X94"=w73:bool, "X95"=w74:bool, "X96"=w75:bool, "X97"=w76:bool, "X98"=w77:bool, "X99"=w78:bool, "X100"=w79:bool, "X101"=w80:bool, "X102"=w81:bool, "X103"=w82:bool, "X104"=w83:bool, "X105"=w84:bool, "X106"=w85:bool, "X107"=w86:bool, "X108"=w87:bool, "X109"=w88:bool, "X110"=w89:bool, "X111"=w90:bool, "X112"=w91:bool, "X113"=w92:bool, "X114"=w93:bool, "X115"=w94:bool, "X116"=w95:bool, "X117"=w96:bool, "X118"=w97:bool, "X119"=w98:bool, "X120"=w99:bool, "X121"=w100:bool, "X122"=w101:bool, "X123"=w102:bool, "X124"=w103:bool, "X125"=w104:bool, "X126"=w105:bool, "X127"=w106:bool)  [unwired: 1 in, 1 out]
  n12 = property class="RtdeIntRegistersValue"(reference=w505) -> (reference out=w9:refnum<k24>, "X0"=w504:i32, "X1"=w503:i32, "X2"=w502:i32, "X3"=w501:i32, "X4"=w500:i32, "X5"=w499:i32, "X6"=w498:i32, "X7"=w497:i32, "X8"=w496:i32, "X9"=w495:i32, "X10"=w494:i32, "X11"=w493:i32, "X12"=w492:i32, "X13"=w491:i32, "X14"=w490:i32, "X15"=w489:i32, "X16"=w488:i32, "X17"=w487:i32, "X18"=w486:i32, "X19"=w485:i32, "X20"=w484:i32, "X21"=w483:i32, "X22"=w482:i32, "X23"=w481:i32, "X24"=w480:i32, "X25"=w479:i32, "X26"=w478:i32, "X27"=w477:i32, "X28"=w476:i32, "X29"=w475:i32, "X30"=w474:i32, "X31"=w473:i32, "X32"=w472:i32, "X33"=w471:i32, "X34"=w470:i32, "X35"=w469:i32, "X36"=w468:i32, "X37"=w467:i32, "X38"=w466:i32, "X39"=w465:i32, "X40"=w464:i32, "X41"=w463:i32, "X42"=w462:i32, "X43"=w461:i32, "X44"=w460:i32, "X45"=w459:i32, "X46"=w458:i32, "X47"=w457:i32)  [unwired: 1 in, 1 out]
  n13 = property class="JointsDoubleValues"(reference=w34) -> (reference out=w30:refnum<k24>, "Base"=w35:dbl, "Elbow"=w36:dbl, "Shoulder"=w37:dbl, "Wrist1"=w38:dbl, "Wrist2"=w39:dbl, "Wrist3"=w40:dbl)  [unwired: 1 in, 1 out]
  n14 = property class="JointsDoubleValues"(reference=w41) -> (reference out=w29:refnum<k24>, "Base"=w121:dbl, "Elbow"=w122:dbl, "Shoulder"=w123:dbl, "Wrist1"=w124:dbl, "Wrist2"=w125:dbl, "Wrist3"=w126:dbl)  [unwired: 1 in, 1 out]
  n15 = property class="JointsDoubleValues"(reference=w113) -> (reference out=w28:refnum<k24>, "Base"=w107:dbl, "Elbow"=w108:dbl, "Shoulder"=w109:dbl, "Wrist1"=w110:dbl, "Wrist2"=w111:dbl, "Wrist3"=w112:dbl)  [unwired: 1 in, 1 out]
  n16 = property class="JointsDoubleValues"(reference=w120) -> (reference out=w27:refnum<k24>, "Base"=w114:dbl, "Elbow"=w115:dbl, "Shoulder"=w116:dbl, "Wrist1"=w117:dbl, "Wrist2"=w118:dbl, "Wrist3"=w119:dbl)  [unwired: 1 in, 1 out]
  n17 = property class="JointsDoubleValues"(reference=w393) -> (reference out=w17:refnum<k24>, "Base"=w387:dbl, "Elbow"=w388:dbl, "Shoulder"=w389:dbl, "Wrist1"=w390:dbl, "Wrist2"=w391:dbl, "Wrist3"=w392:dbl)  [unwired: 1 in, 1 out]
  n18 = property class="JointsDoubleValues"(reference=w402) -> (reference out=w14:refnum<k24>, "Base"=w401:dbl, "Elbow"=w400:dbl, "Shoulder"=w399:dbl, "Wrist1"=w398:dbl, "Wrist2"=w397:dbl, "Wrist3"=w396:dbl)  [unwired: 1 in, 1 out]
  n19 = property class="JointsDoubleValues"(reference=w545) -> (reference out=w8:refnum<k24>, "Base"=w539:dbl, "Elbow"=w540:dbl, "Shoulder"=w541:dbl, "Wrist1"=w542:dbl, "Wrist2"=w543:dbl, "Wrist3"=w544:dbl)  [unwired: 1 in, 1 out]
  n20 = property class="JointsDoubleValues"(reference=w546) -> (reference out=w7:refnum<k24>, "Base"=w538:dbl, "Elbow"=w537:dbl, "Shoulder"=w536:dbl, "Wrist1"=w535:dbl, "Wrist2"=w534:dbl, "Wrist3"=w533:dbl)  [unwired: 1 in, 1 out]
  n21 = property class="JointsDoubleValues"(reference=w152) -> (reference out=w6:refnum<k24>, "Base"=w134:dbl, "Elbow"=w135:dbl, "Shoulder"=w136:dbl, "Wrist1"=w137:dbl, "Wrist2"=w138:dbl, "Wrist3"=w139:dbl)  [unwired: 1 in, 1 out]
  n22 = property class="JointsDoubleValues"(reference=w153) -> (reference out=w5:refnum<k24>, "Base"=w140:dbl, "Elbow"=w141:dbl, "Shoulder"=w142:dbl, "Wrist1"=w143:dbl, "Wrist2"=w144:dbl, "Wrist3"=w145:dbl)  [unwired: 1 in, 1 out]
  n23 = property class="JointsDoubleValues"(reference=w154) -> (reference out=w4:refnum<k24>, "Base"=w146:dbl, "Elbow"=w147:dbl, "Shoulder"=w148:dbl, "Wrist1"=w149:dbl, "Wrist2"=w150:dbl, "Wrist3"=w151:dbl)  [unwired: 1 in, 1 out]
  n24 = property class="JointsIntValues"(reference=w127) -> (reference out=w16:refnum<k24>, "Base"=w128:i32, "Elbow"=w129:i32, "Shoulder"=w130:i32, "Wrist1"=w131:i32, "Wrist2"=w132:i32, "Wrist3"=w133:i32)  [unwired: 1 in, 1 out]
  n25 = property class="Vector3D"(reference=w190) -> (reference out=w23:refnum<k24>, "X"=w191:dbl, "Y"=w192:dbl, "Z"=w193:dbl)  [unwired: 1 in, 1 out]
  n26 = property class="Vector3D"(reference=w196) -> (reference out=w22:refnum<k24>, "X"=w197:dbl, "Y"=w198:dbl, "Z"=w199:dbl)  [unwired: 1 in, 1 out]
  n27 = property class="Vector3D"(reference=w201) -> (reference out=w21:refnum<k24>, "X"=w202:dbl, "Y"=w203:dbl, "Z"=w204:dbl)  [unwired: 1 in, 1 out]
  n28 = property class="Vector3D"(reference=w510) -> (reference out=w11:refnum<k24>, "X"=w507:dbl, "Y"=w508:dbl, "Z"=w509:dbl)  [unwired: 1 in, 1 out]
  n29 = property class="Pose"(reference=w166) -> (reference out=w25:refnum<k24>, "X"=w167:dbl, "Y"=w168:dbl, "Z"=w169:dbl, "Rx"=w170:dbl, "Ry"=w171:dbl, "Rz"=w172:dbl)  [unwired: 1 in, 1 out]
  n30 = property class="Pose"(reference=w188) -> (reference out=w24:refnum<k24>, "X"=w182:dbl, "Y"=w183:dbl, "Z"=w184:dbl, "Rx"=w185:dbl, "Ry"=w186:dbl, "Rz"=w187:dbl)  [unwired: 1 in, 1 out]
  n31 = property class="Pose"(reference=w565) -> (reference out=w3:refnum<k24>, "X"=w553:dbl, "Y"=w554:dbl, "Z"=w555:dbl, "Rx"=w556:dbl, "Ry"=w557:dbl, "Rz"=w558:dbl)  [unwired: 1 in, 1 out]
  n32 = property class="Pose"(reference=w566) -> (reference out=w2:refnum<k24>, "X"=w559:dbl, "Y"=w560:dbl, "Z"=w561:dbl, "Rx"=w562:dbl, "Ry"=w563:dbl, "Rz"=w564:dbl)  [unwired: 1 in, 1 out]
  n33 = Close Reference(reference=w11) -> ()  [unwired: 1 in, 1 out]
  n34 = Close Reference(reference=w4) -> ()  [unwired: 1 in, 1 out]
  n35 = Close Reference(reference=w3) -> ()  [unwired: 1 in, 1 out]
  n36 = Close Reference(reference=w2) -> ()  [unwired: 1 in, 1 out]
  n37 = Close Reference(reference=w13) -> ()  [unwired: 1 in, 1 out]
  n38 = Close Reference(reference=w7) -> ()  [unwired: 1 in, 1 out]
  n39 = Close Reference(reference=w5) -> ()  [unwired: 1 in, 1 out]
  n40 = Close Reference(reference=w6) -> ()  [unwired: 1 in, 1 out]
  n41 = Close Reference(reference=w14) -> ()  [unwired: 1 in, 1 out]
  n42 = Close Reference(reference=w12) -> ()  [unwired: 1 in, 1 out]
  n43 = Close Reference(reference=w15) -> ()  [unwired: 1 in, 1 out]
  n44 = Close Reference(reference=w23) -> ()  [unwired: 1 in, 1 out]
  n45 = Close Reference(reference=w8) -> ()  [unwired: 1 in, 1 out]
  n46 = Close Reference(reference=w21) -> ()  [unwired: 1 in, 1 out]
  n47 = Close Reference(reference=w24) -> ()  [unwired: 1 in, 1 out]
  n48 = Close Reference(reference=w17) -> ()  [unwired: 1 in, 1 out]
  n49 = Close Reference(reference=w16) -> ()  [unwired: 1 in, 1 out]
  n50 = Close Reference(reference=w10) -> ()  [unwired: 1 in, 1 out]
  n51 = Close Reference(reference=w27) -> ()  [unwired: 1 in, 1 out]
  n52 = Close Reference(reference=w22) -> ()  [unwired: 1 in, 1 out]
  n53 = Close Reference(reference=w9) -> ()  [unwired: 1 in, 1 out]
  n54 = Close Reference(reference=w25) -> ()  [unwired: 1 in, 1 out]
  n55 = Close Reference(reference=w29) -> ()  [unwired: 1 in, 1 out]
  n56 = Close Reference(reference=w19) -> ()  [unwired: 1 in, 1 out]
  n57 = Close Reference(reference=w28) -> ()  [unwired: 1 in, 1 out]
  n58 = Close Reference(reference=w18) -> ()  [unwired: 1 in, 1 out]
  n59 = Close Reference(reference=w20) -> ()  [unwired: 1 in, 1 out]
  n60 = Close Reference(reference=w30) -> ()  [unwired: 1 in, 1 out]
  n61 = Close Reference(reference=w26) -> ()  [unwired: 1 in, 1 out]
  n62 = Bundle("Base"=w35, "Elbow"=w36, "Shoulder"=w37, "Wrist1"=w38, "Wrist2"=w39, "Wrist3"=w40) -> (w155:T2)  [unwired: 1 in]
  n63 = Bundle("Base"=w121, "Elbow"=w122, "Shoulder"=w123, "Wrist1"=w124, "Wrist2"=w125, "Wrist3"=w126) -> (w159:T2)  [unwired: 1 in]
  n64 = Bundle("Base"=w107, "Elbow"=w108, "Shoulder"=w109, "Wrist1"=w110, "Wrist2"=w111, "Wrist3"=w112) -> (w162:T2)  [unwired: 1 in]
  n65 = Bundle("Base"=w114, "Elbow"=w115, "Shoulder"=w116, "Wrist1"=w117, "Wrist2"=w118, "Wrist3"=w119) -> (w163:T2)  [unwired: 1 in]
  n66 = Bundle("X"=w178, "Y"=w177, "Z"=w176, "Rx"=w175, "Ry"=w174, "Rz"=w173) -> (w180:T3)  [unwired: 1 in]
  n67 = Bundle("X"=w167, "Y"=w168, "Z"=w169, "Rx"=w170, "Ry"=w171, "Rz"=w172) -> (w181:T3)  [unwired: 1 in]
  n68 = Bundle("X"=w182, "Y"=w183, "Z"=w184, "Rx"=w185, "Ry"=w186, "Rz"=w187) -> (w189:T3)  [unwired: 1 in]
  n69 = Bundle("X"=w191, "Y"=w192, "Z"=w193) -> (w194:cluster{"X":dbl, "Y":dbl, "Z":dbl})  [unwired: 1 in]
  n70 = Bundle("X"=w197, "Y"=w198, "Z"=w199) -> (w200:cluster{"X":dbl, "Y":dbl, "Z":dbl})  [unwired: 1 in]
  n71 = Bundle("X"=w202, "Y"=w203, "Z"=w204) -> (w205:cluster{"X":dbl, "Y":dbl, "Z":dbl})  [unwired: 1 in]
  n72 = Bundle("X"=w210, "Y"=w211, "Z"=w212, "Rx"=w213, "Ry"=w214, "Rz"=w215) -> (w217:T3)  [unwired: 1 in]
  n73 = Bundle("X64"=w281, "X65"=w280, "X66"=w279, "X67"=w278, "X68"=w277, "X69"=w276, "X70"=w275, "X71"=w274, "X72"=w273, "X73"=w272, "X74"=w271, "X75"=w270, "X76"=w269, "X77"=w268, "X78"=w267, "X79"=w266, "X80"=w265, "X81"=w264, "X82"=w263, "X83"=w262, "X84"=w261, "X85"=w260, "X86"=w259, "X87"=w258, "X88"=w257, "X89"=w256, "X90"=w255, "X91"=w254, "X92"=w253, "X93"=w252, "X94"=w251, "X95"=w250, "X96"=w249, "X97"=w248, "X98"=w247, "X99"=w246, "X100"=w245, "X101"=w244, "X102"=w243, "X103"=w242, "X104"=w241, "X105"=w240, "X106"=w239, "X107"=w238, "X108"=w237, "X109"=w236, "X110"=w235, "X111"=w234, "X112"=w233, "X113"=w232, "X114"=w231, "X115"=w230, "X116"=w229, "X117"=w228, "X118"=w227, "X119"=w226, "X120"=w225, "X121"=w224, "X122"=w223, "X123"=w222, "X124"=w221, "X125"=w220, "X126"=w219, "X127"=w218) -> (w283:T4)  [unwired: 1 in]
  n74 = Bundle("X0"=w285, "X1"=w286, "X2"=w287, "X3"=w288, "X4"=w289, "X5"=w290, "X6"=w291, "X7"=w292, "X8"=w293, "X9"=w294, "X10"=w295, "X11"=w296, "X12"=w297, "X13"=w298, "X14"=w299, "X15"=w300, "X16"=w301, "X17"=w302, "X18"=w303, "X19"=w304, "X20"=w305, "X21"=w306, "X22"=w307, "X23"=w308, "X24"=w309, "X25"=w310, "X26"=w311, "X27"=w312, "X28"=w313, "X29"=w314, "X30"=w315, "X31"=w316, "X32"=w317, "X33"=w318, "X34"=w319, "X35"=w320, "X36"=w321, "X37"=w322, "X38"=w323, "X39"=w324, "X40"=w325, "X41"=w326, "X42"=w327, "X43"=w328, "X44"=w329, "X45"=w330, "X46"=w331, "X47"=w332) -> (w335:T5)  [unwired: 1 in]
  n75 = Bundle("Base"=w387, "Elbow"=w388, "Shoulder"=w389, "Wrist1"=w390, "Wrist2"=w391, "Wrist3"=w392) -> (w394:T2)  [unwired: 1 in]
  n76 = Bundle("Base"=w128, "Elbow"=w129, "Shoulder"=w130, "Wrist1"=w131, "Wrist2"=w132, "Wrist3"=w133) -> (w395:T6)  [unwired: 1 in]
  n77 = Bundle("X0"=w336, "X1"=w337, "X2"=w338, "X3"=w339, "X4"=w340, "X5"=w341, "X6"=w342, "X7"=w343, "X8"=w344, "X9"=w345, "X10"=w346, "X11"=w347, "X12"=w348, "X13"=w349, "X14"=w350, "X15"=w351, "X16"=w352, "X17"=w353, "X18"=w354, "X19"=w355, "X20"=w356, "X21"=w357, "X22"=w358, "X23"=w359, "X24"=w360, "X25"=w361, "X26"=w362, "X27"=w363, "X28"=w364, "X29"=w365, "X30"=w366, "X31"=w367, "X32"=w368, "X33"=w369, "X34"=w370, "X35"=w371, "X36"=w372, "X37"=w373, "X38"=w374, "X39"=w375, "X40"=w376, "X41"=w377, "X42"=w378, "X43"=w379, "X44"=w380, "X45"=w381, "X46"=w382, "X47"=w383) -> (w385:T7)  [unwired: 1 in]
  n78 = Bundle("Base"=w401, "Elbow"=w400, "Shoulder"=w399, "Wrist1"=w398, "Wrist2"=w397, "Wrist3"=w396) -> (w403:T2)  [unwired: 1 in]
  n79 = Bundle("X64"=w43, "X65"=w44, "X66"=w45, "X67"=w46, "X68"=w47, "X69"=w48, "X70"=w49, "X71"=w50, "X72"=w51, "X73"=w52, "X74"=w53, "X75"=w54, "X76"=w55, "X77"=w56, "X78"=w57, "X79"=w58, "X80"=w59, "X81"=w60, "X82"=w61, "X83"=w62, "X84"=w63, "X85"=w64, "X86"=w65, "X87"=w66, "X88"=w67, "X89"=w68, "X90"=w69, "X91"=w70, "X92"=w71, "X93"=w72, "X94"=w73, "X95"=w74, "X96"=w75, "X97"=w76, "X98"=w77, "X99"=w78, "X100"=w79, "X101"=w80, "X102"=w81, "X103"=w82, "X104"=w83, "X105"=w84, "X106"=w85, "X107"=w86, "X108"=w87, "X109"=w88, "X110"=w89, "X111"=w90, "X112"=w91, "X113"=w92, "X114"=w93, "X115"=w94, "X116"=w95, "X117"=w96, "X118"=w97, "X119"=w98, "X120"=w99, "X121"=w100, "X122"=w101, "X123"=w102, "X124"=w103, "X125"=w104, "X126"=w105, "X127"=w106) -> (w404:T4)  [unwired: 1 in]
  n80 = Bundle("X0"=w407, "X1"=w408, "X2"=w409, "X3"=w410, "X4"=w411, "X5"=w412, "X6"=w413, "X7"=w414, "X8"=w415, "X9"=w416, "X10"=w417, "X11"=w418, "X12"=w419, "X13"=w420, "X14"=w421, "X15"=w422, "X16"=w423, "X17"=w424, "X18"=w425, "X19"=w426, "X20"=w427, "X21"=w428, "X22"=w429, "X23"=w430, "X24"=w431, "X25"=w432, "X26"=w433, "X27"=w434, "X28"=w435, "X29"=w436, "X30"=w437, "X31"=w438, "X32"=w439, "X33"=w440, "X34"=w441, "X35"=w442, "X36"=w443, "X37"=w444, "X38"=w445, "X39"=w446, "X40"=w447, "X41"=w448, "X42"=w449, "X43"=w450, "X44"=w451, "X45"=w452, "X46"=w453, "X47"=w454) -> (w456:T5)  [unwired: 1 in]
  n81 = Bundle("X"=w507, "Y"=w508, "Z"=w509) -> (w512:cluster{"X":dbl, "Y":dbl, "Z":dbl})  [unwired: 1 in]
  n82 = Bundle("X"=w513, "Y"=w514, "Z"=w515, "Rx"=w516, "Ry"=w517, "Rz"=w518) -> (w520:T3)  [unwired: 1 in]
  n83 = Bundle("X0"=w504, "X1"=w503, "X2"=w502, "X3"=w501, "X4"=w500, "X5"=w499, "X6"=w498, "X7"=w497, "X8"=w496, "X9"=w495, "X10"=w494, "X11"=w493, "X12"=w492, "X13"=w491, "X14"=w490, "X15"=w489, "X16"=w488, "X17"=w487, "X18"=w486, "X19"=w485, "X20"=w484, "X21"=w483, "X22"=w482, "X23"=w481, "X24"=w480, "X25"=w479, "X26"=w478, "X27"=w477, "X28"=w476, "X29"=w475, "X30"=w474, "X31"=w473, "X32"=w472, "X33"=w471, "X34"=w470, "X35"=w469, "X36"=w468, "X37"=w467, "X38"=w466, "X39"=w465, "X40"=w464, "X41"=w463, "X42"=w462, "X43"=w461, "X44"=w460, "X45"=w459, "X46"=w458, "X47"=w457) -> (w506:T7)  [unwired: 1 in]
  n84 = Bundle("Base"=w539, "Elbow"=w540, "Shoulder"=w541, "Wrist1"=w542, "Wrist2"=w543, "Wrist3"=w544) -> (w547:T2)  [unwired: 1 in]
  n85 = Bundle("Base"=w538, "Elbow"=w537, "Shoulder"=w536, "Wrist1"=w535, "Wrist2"=w534, "Wrist3"=w533) -> (w548:T2)  [unwired: 1 in]
  n86 = Bundle("Base"=w134, "Elbow"=w135, "Shoulder"=w136, "Wrist1"=w137, "Wrist2"=w138, "Wrist3"=w139) -> (w549:T2)  [unwired: 1 in]
  n87 = Bundle("Base"=w140, "Elbow"=w141, "Shoulder"=w142, "Wrist1"=w143, "Wrist2"=w144, "Wrist3"=w145) -> (w550:T2)  [unwired: 1 in]
  n88 = Bundle("Base"=w146, "Elbow"=w147, "Shoulder"=w148, "Wrist1"=w149, "Wrist2"=w150, "Wrist3"=w151) -> (w551:T2)  [unwired: 1 in]
  n89 = Bundle("X"=w553, "Y"=w554, "Z"=w555, "Rx"=w556, "Ry"=w557, "Rz"=w558) -> (w567:T3)  [unwired: 1 in]
  n90 = Bundle("X"=w559, "Y"=w560, "Z"=w561, "Rx"=w562, "Ry"=w563, "Rz"=w564) -> (w568:T3)  [unwired: 1 in]
  n91 = Bundle(w155, "ActualDigitalInputBits"=w156, "ActualDigitalOutputBits"=w157, "ActualExecutionTime"=w158, w159, "ActualMainVoltage"=w160, "ActualMomentum"=w161, w162, w163, "ActualRobotCurrent"=w164, "ActualRobotVoltage"=w165, w180, w181, w189, w194, "AnalogIOTypes"=w195, w200, w205, "Euromap67_24VCurrent"=w206, "Euromap67_24VVoltage"=w207, "Euromap67InputBits"=w208, "Euromap67OutputBits"=w209, w217, w283, "InputBitRegisters0To31"=w334, "InputBitRegisters32To63"=w333, w335, w385, "IOCurrent"=w386, w394, w395, w403, w404, "OutputBitRegisters0To31"=w405, "OutputBitRegisters32To63"=w406, w456, w506, "Payload"=w511, w512, w520, "RobotMode"=w521, "RobotStatusBits"=w522, "RuntimeState"=w523, "SafetyMode"=w524, "SafetyStatus"=w525, "SafetyStatusBits"=w526, "ScriptControlLine"=w527, "SpeedScaling"=w528, "StandardAnalogInput0"=w529, "StandardAnalogInput1"=w530, "StandardAnalogOutput0"=w531, "StandardAnalogOutput1"=w532, w547, w548, w549, w550, w551, "TargetSpeedFraction"=w552, w567, w568, "TcpForceScalar"=w569, "Timestamp"=w570, "ToolAnalogInput0"=w571, "ToolAnalogInput1"=w572, "ToolAnalogInputTypes"=w573, "ToolDigitalOutput0mode"=w574, "ToolDigitalOutput1Mode"=w575, "ToolMode"=w576, "ToolOutputCurrent"=w577, "ToolOutputMode"=w578, "ToolOutputVoltage"=w579, "ToolTemperature"=w580) -> (→"Data":T8)  [unwired: 1 in]
